vi "Quack.vi"(8 "error in (no error)":errorcluster, 11 "TurkeyAdapter in":refnum<class "TurkeyAdapter.lvclass">) -> (0 "error out":errorcluster, 2 "Quack":string, 3 "TurkeyAdapter out":refnum<class "TurkeyAdapter.lvclass">)   [LabVIEW 2013, in "TurkeyAdapter.lvclass"]
uses:
  TurkeyAdapter.lvclass
  TurkeyAdapter.lvclass/TurkeyAdapter.ctl
  Turkey.lvclass/Turkey.lvclass
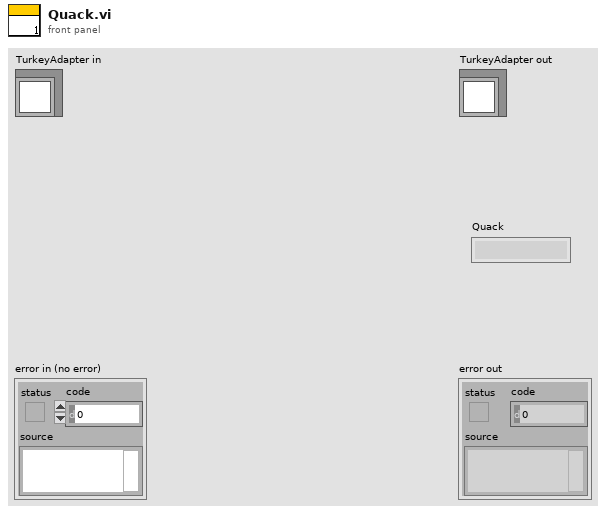
[diagram p1: front panel]
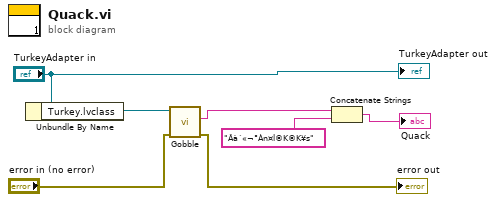
[diagram p0: block diagram]
diagram:
  n1 = Unbundle By Name("TurkeyAdapter in") -> ("Turkey.lvclass"=w4:refnum<class "Turkey.lvclass">)
  n2 = call-dynamic "Gobble.vi"("error in (no error)"="error in (no error)", "Turkey in"=w4) -> ("error out"=→"error out":errorcluster, "Gobble"=w1:string)  [unwired: 7 in, 1 out]
  n3 = Concatenate Strings(w1, "Âà´«¬°Àn¤l©K©K¥s" ("string")) -> (→"Quack":string)
  "TurkeyAdapter out" <- "TurkeyAdapter in"
